vi "rqcBob ServiceNET Read Command.vi"(8 "error in":errorcluster, 9 "timeout ms (50)":i32=50, 11 "rqcBob ServiceNET in":T2) -> (0 "error out":errorcluster, 1 "cmd valid":bool, 2 "command":T1=enum."READY", 3 "rqcBob ServiceNET out":T2)   [LabVIEW 2018]
uses:
  Custom Controls/rqcBob ServiceNET control.ctl
  Custom Controls/rqc ServiceNET command.ctl
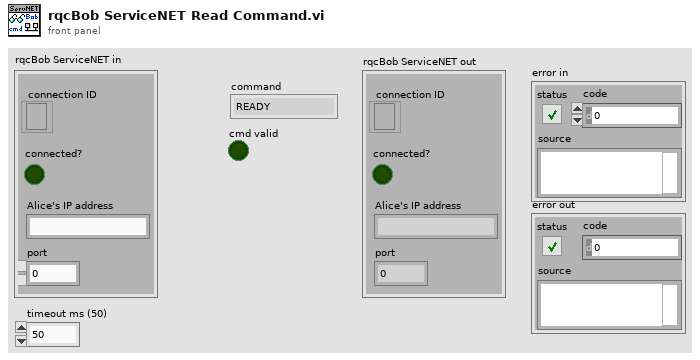
[diagram p1: front panel]
types:
  T1 = typedef "rqc ServiceNET command.ctl" = enum8{"NONE", "READY", "START", "PING", "SEND KEY", "WRITE KEY", "WRITE AND SAVE KEY"}
  T2 = typedef "rqcBob ServiceNET control.ctl" = cluster{"connection ID":refnum<k5>, "connected?":bool, "Alice's IP address":string, "port":u16}
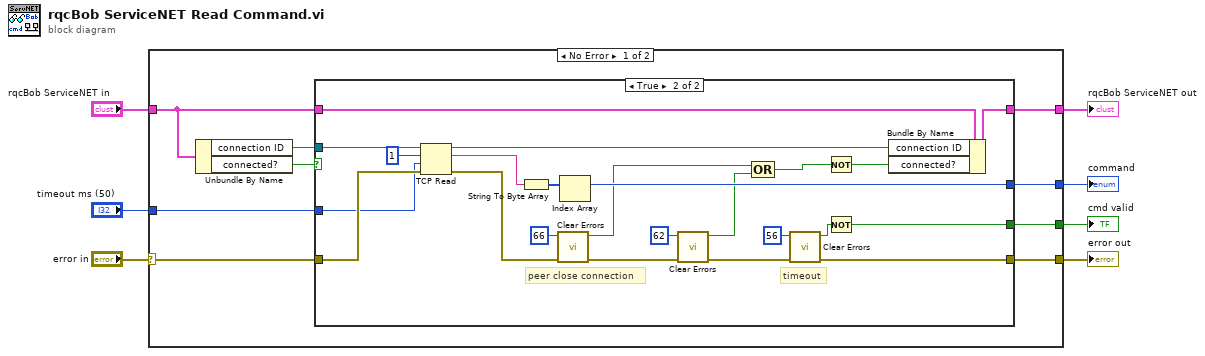
[diagram p0: block diagram]
diagram:
  n1 = case shown="No Error" "error in" {
    selector: "error in" -> [w14 w43]
    tunnel: "rqcBob ServiceNET in" -> [w12 w42]
    tunnel: [w13 w43] -> w5
    tunnel: [w11 w42] -> w4
    tunnel: [w10 _] -> w3
    tunnel: [w9 _] -> w2
    tunnel: "timeout ms (50)" -> [w8 _]
    frame No Error {
      n2 = Unbundle By Name(w12) -> ("connection ID"=w15:refnum<k5>, "connected?"=w16:bool)
      n3 = case shown="True" w16 {
        tunnel: w15 -> [_ w39]
        tunnel: w14 -> [w18 w37]
        tunnel: [w18 w29] -> w13
        tunnel: [w17 w40] -> w11
        tunnel: w12 -> [w17 w41]
        tunnel: [_ w33] -> w10
        tunnel: [_ w26] -> w9
        tunnel: w8 -> [_ w19]
        frame False {
        }
        frame True {
          # "peer close connection"
          # "timeout"
          n4 = TCP Read(connection ID=w39, bytes to read=1, error in (no error)=w37, 9:w19) -> (connection ID out=w38:refnum<k5>, data out=w35:string, error out=w28:errorcluster)  [unwired: 1 in]
          n5 = String To Byte Array(string=w35) -> (unsigned byte array=w34:u8[])
          n6 = call <vilib>:"Clear Errors.vi"("error in (no error)"=w28, "specific error code to clear (0: all)"=66) -> ("error out"=w25:errorcluster, "specific error cleared?"=w22:bool)  [unwired: 4 in]
          n7 = Index Array(array=w34) -> (element=w33:u8)  [unwired: 1 in]
          n8 = call <vilib>:"Clear Errors.vi"("error in (no error)"=w25, "specific error code to clear (0: all)"=62) -> ("error out"=w24:errorcluster, "specific error cleared?"=w20:bool)  [unwired: 4 in]
          n9 = Compound Arithmetic op=OR(w22, w20) -> (w21:bool)
          n10 = call <vilib>:"Clear Errors.vi"("error in (no error)"=w24, "specific error code to clear (0: all)"=56) -> ("error out"=w29:errorcluster, "specific error cleared?"=w27:bool)  [unwired: 4 in]
          n11 = Not(x=w21) -> (.not. x?=w30:bool)
          n12 = Not(x=w27) -> (.not. x?=w26:bool)
          n13 = Bundle By Name(cluster=w41, "connection ID"=w38, "connected?"=w30) -> (w40:T2)
        }
      }
    }
    frame Error {
    }
  }
  "error out" <- w5
  "rqcBob ServiceNET out" <- w4
  "command" <- w3
  "cmd valid" <- w2
